vi "update.vi"(8 "error in (no error)":errorcluster, 9 "Actuate Settings":T1, 10 "ILC in":refnum<class "ILC.lvclass">, 11 "SingleCylinderActuator in":refnum<class "SingleCylinderActuator.lvclass">) -> (0 "error out":errorcluster, 2 "ILC out":refnum<class "ILC.lvclass">, 3 "SingleCylinderActuator out":refnum<class "SingleCylinderActuator.lvclass">)   [LabVIEW 2015, in "SingleCylinderActuator.lvclass"]
uses:
  SingleCylinderActuator.lvclass
  Typedefs/Actuate Settings.ctl
  Typedefs/ControlMode.ctl
  <userlib>/Common/ILC/ILC/ILC.lvclass
  SingleCylinderActuator.lvclass/SingleCylinderActuator.ctl
  <vilib>/addons/control/pid/pid.llb/PID (DBL).vi
  ActuatorCylinder/IActuatorCylinder/IActuatorCylinder.lvclass
  <vilib>/addons/control/pid/NI_PID_pid.lvlib
  Calculators/ForceToPressureServoVoltage/ForceToPressureServoVoltage.lvclass
  Typedefs/FAMTTypedefs.lvlib
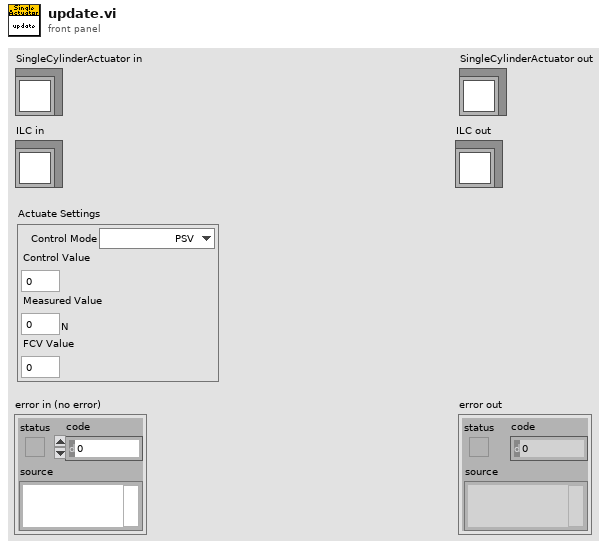
[diagram p1: front panel]
types:
  T1 = typedef "FAMTTypedefs.lvlib/Actuate Settings.ctl" = cluster{"Control Mode":T2, "Control Value":dbl, "Measured Value":dbl[unit], "FCV Value":dbl}
  T2 = typedef "FAMTTypedefs.lvlib/ControlMode.ctl" = enum16{"PSV", "FCV", "Both"}
  T3 = cluster{"proportional gain (Kc)":dbl, "integral time (Ti, min)":dbl, "derivative time (Td, min)":dbl}
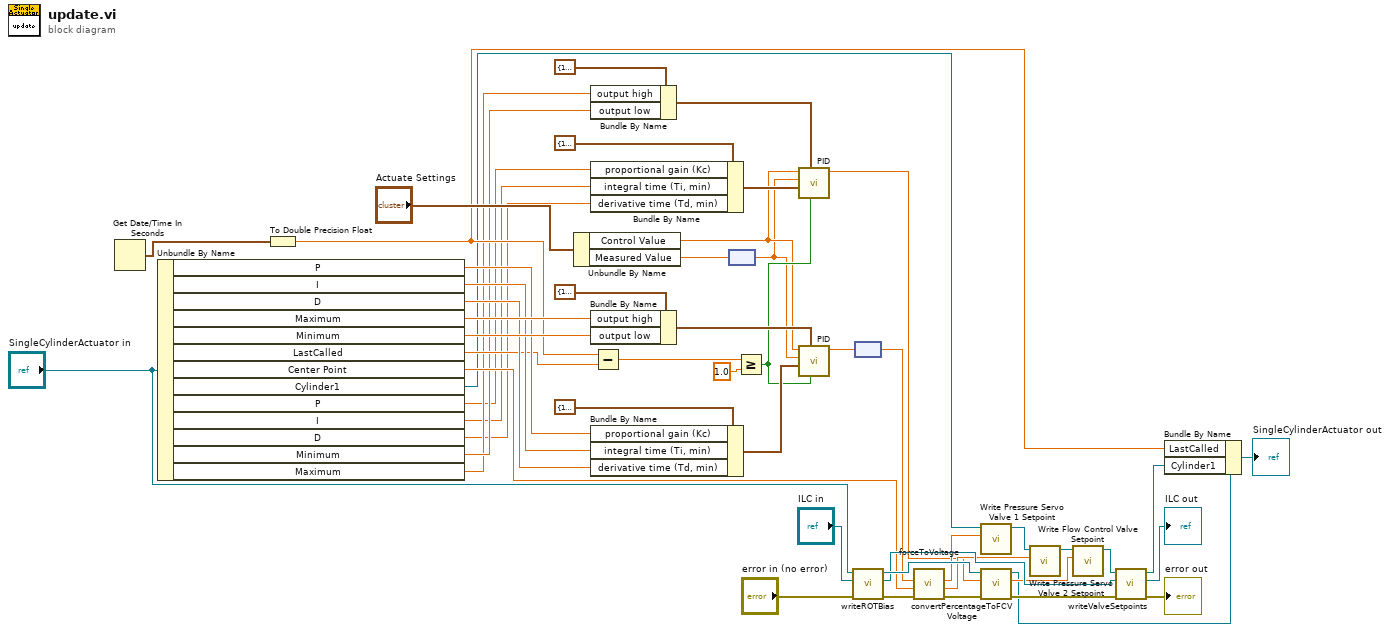
[diagram p0: block diagram]
diagram:
  n1 = Get Date/Time In Seconds() -> (seconds since 1Jan1904=w41:timestamp)
  n2 = Unbundle By Name("SingleCylinderActuator in") -> ("P"=w46:dbl, "I"=w45:dbl, "D"=w44:dbl, "Maximum"=w50:dbl, "Minimum"=w49:dbl, "LastCalled"=w40:dbl, "Center Point"=w27:dbl[unit], "Cylinder1"=w22:refnum<class "IActuatorCylinder.lvclass">, "P"=w7:dbl, "I"=w6:dbl, "D"=w5:dbl, "Minimum"=w9:dbl, "Maximum"=w8:dbl)
  n3 = To Double Precision Float(number=w41) -> (double precision float=w37:dbl)
  n4 = Unbundle By Name("Actuate Settings") -> ("Control Value"=w3:dbl, "Measured Value"=w42:dbl[unit])
  n5 = Bundle By Name(cluster=cluster{"output high":dbl, "output low":dbl} {"output high"=100.0, "output low"=-100.0} ("output range"), "output high"=w8, "output low"=w9) -> (w4:cluster{"output high":dbl, "output low":dbl})
  n6 = Bundle By Name(cluster=T3 {"proportional gain (Kc)"=1.0, "integral time (Ti, min)"=0.01, "derivative time (Td, min)"=0.0} ("PID gains"), "proportional gain (Kc)"=w7, "integral time (Ti, min)"=w6, "derivative time (Td, min)"=w5) -> (w12:T3)
  n7 = Bundle By Name(cluster=cluster{"output high":dbl, "output low":dbl} {"output high"=100.0, "output low"=-100.0} ("output range"), "output high"=w50, "output low"=w49) -> (w51:cluster{"output high":dbl, "output low":dbl})
  n8 = Bundle By Name(cluster=T3 {"proportional gain (Kc)"=1.0, "integral time (Ti, min)"=0.01, "derivative time (Td, min)"=0.0} ("PID gains"), "proportional gain (Kc)"=w46, "integral time (Ti, min)"=w45, "derivative time (Td, min)"=w44) -> (w47:T3)
  n9 = Subtract(x=w37, y=w40) -> (x-y=w39:dbl)
  n10 = node(w42) -> (w2:dbl)
  n11 = Greater Or Equal?(x=w39, y=1.0) -> (x >= y?=w11:bool)
  n12 = call-poly <vilib>:"PID.vi"("reinitialize? (F)"=w11, "output range"=w4, "PID gains"=w12, "process variable"=w2, "setpoint"=w3) -> ("output"=w1:dbl)  [unwired: 5 in, 1 out]
  n13 = call-poly <vilib>:"PID.vi"("reinitialize? (F)"=w11, "output range"=w51, "PID gains"=w47, "process variable"=w2, "setpoint"=w3) -> ("output"=w26:dbl)  [unwired: 5 in, 1 out]
  n14 = call "writeROTBias.vi"("error in (no error)"="error in (no error)", "ILC in"="ILC in", "SingleCylinderActuator in"="SingleCylinderActuator in") -> ("error out"=w31:errorcluster, "ILC out"=w34:refnum<class "ILC.lvclass">, "SingleCylinderActuator out"=w36:refnum<class "SingleCylinderActuator.lvclass">)  [unwired: 6 in]
  n15 = node(w26) -> (w25:dbl[unit])
  n16 = call "forceToVoltage.vi"("error in (no error)"=w31, "Center Point"=w27, "Force"=w25) -> ("error out"=w30:errorcluster, "Voltage 2"=w23:dbl[unit], "Voltage 1"=w24:dbl[unit])  [unwired: 5 in, 1 out]
  n17 = call-dynamic "Write Pressure Servo Valve 1 Setpoint.vi"("Pressure Servo Valve 1 Setpoint"=w24, "IActuatorCylinder in"=w22) -> ("IActuatorCylinder out"=w21:refnum<class "IActuatorCylinder.lvclass">)  [unwired: 9 in]
  n18 = call "convertPercentageToFCVVoltage.vi"("error in (no error)"=w30, "Percentage"=w1, "SingleCylinderActuator in"=w36) -> ("error out"=w29:errorcluster, "Voltage"=w20:dbl, "SingleCylinderActuator out"=w16:refnum<class "SingleCylinderActuator.lvclass">)  [unwired: 6 in]
  n19 = call-dynamic "Write Pressure Servo Valve 2 Setpoint.vi"("Pressure Servo Valve 2 Setpoint"=w23, "IActuatorCylinder in"=w21) -> ("IActuatorCylinder out"=w19:refnum<class "IActuatorCylinder.lvclass">)  [unwired: 9 in]
  n20 = call-dynamic "Write Flow Control Valve Setpoint.vi"("Flow Control Valve Setpoint"=w20, "IActuatorCylinder in"=w19) -> ("IActuatorCylinder out"=w18:refnum<class "IActuatorCylinder.lvclass">)  [unwired: 9 in]
  n21 = call-dynamic "writeValveSetpoints.vi"("error in (no error)"=w29, "ILC in"=w34, "IActuatorCylinder in"=w18) -> ("error out"=→"error out":errorcluster, "ILC out"=→"ILC out":refnum<class "ILC.lvclass">, "IActuatorCylinder out"=w14:refnum<class "IActuatorCylinder.lvclass">)  [unwired: 6 in]
  n22 = Bundle By Name(cluster=w16, "LastCalled"=w37, "Cylinder1"=w14) -> (→"SingleCylinderActuator out":refnum<class "SingleCylinderActuator.lvclass">)
